vi "Find Pointers by Type.vi"(8 "error in (no error)":errorcluster, 10 "Exclusion List":string[](array[string]), 11 "For Loop Dialog in":refnum<class "For Loop Dialog.lvclass">) -> (0 "error out":errorcluster, 1 "Valid Pointer Names":string[](array[string]), 2 "Valid Pointer IDs":string[](array[string]), 3 "For Loop Dialog out":refnum<class "For Loop Dialog.lvclass">)   [LabVIEW 2017, in "For Loop Dialog.lvclass"]
uses:
  For Loop Dialog.lvclass
  D:/Test-executive-builder/Source/Test Executive Builder Dialogs/ITest Executive Builder Dialog/ITest Executive Builder Dialog.lvclass
  Data Type Handler/Test Executive Builder Data Type Handler.lvclass
  ITest Executive Builder Dialog/ITest Executive Builder Dialog.lvclass/ITest Executive Builder Dialog.ctl
  fa25b816-3366-474b-a896-5c13e2aa05e5.vi
  fa25b816-3366-474b-a896-5c13e2aa05e5.vi/6ced9730-0ebc-45dd-8907-f88a5c37d4f4.vi
  ITest Executive Builder Dialog/Read Test Executive Ref.vi
  ITest Executive Builder Dialog/Read GUID.vi
  ITest Executive Builder Dialog/Read Data Type Handler Type.vi
  <vilib>/Utility/error.llb/Clear Errors.vi
  <vilib>/gpm_packages/@cs/test-executive/Source/Test Executive/TestExecutive Ref/Get Name.vi
  <vilib>/gpm_packages/@cs/test-executive/Source/Test Executive/ITestExecutive/ITest Executive.lvclass
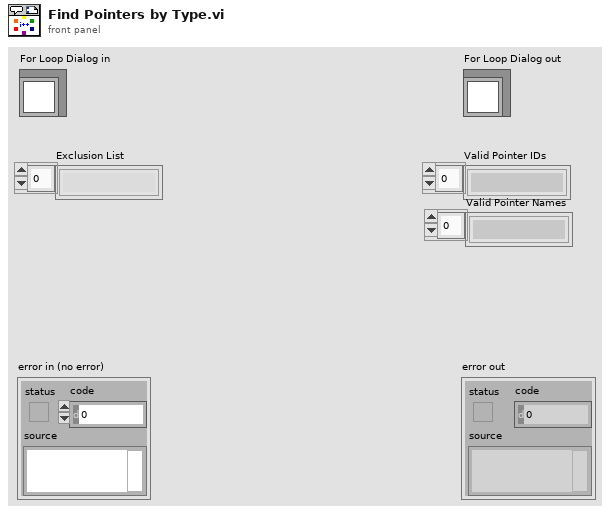
[diagram p1: front panel]
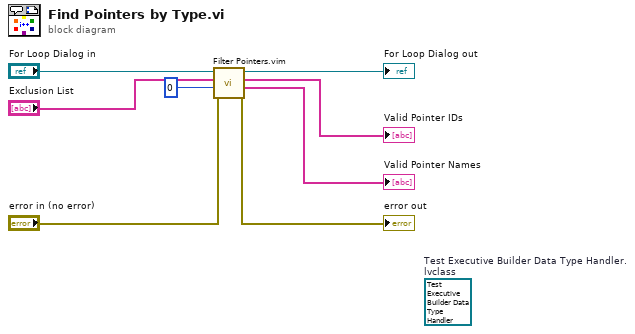
[diagram p0: block diagram]
diagram:
  (unwired) refnum<class "Test Executive Builder Data Type Handler.lvclass"> refnum  # Test Executive Builder Data Type Handler.lvclass
  n1 = call "Filter Pointers.vim"("error in (no error)"="error in (no error)", "Type"=0, "Exclusion List"="Exclusion List", "ITest Executive Builder Dialog in"="For Loop Dialog in") -> ("error out"=→"error out":errorcluster, "Valid Pointer Names"=→"Valid Pointer Names":string[], "Valid Pointer IDs"=→"Valid Pointer IDs":string[], "ITest Executive Builder Dialog out"=→"For Loop Dialog out":refnum<class "For Loop Dialog.lvclass">)  [unwired: 4 in]
